vi "GetFirstProcessModule.vi"(7 "originator":string, 8 "error in (no error)":errorcluster, 9 "data":T2, 10 "type":T1, 11 "Qbus in":refnum<class "Qbus.lvclass">) -> (0 "error out":errorcluster, 3 "Qbus out":refnum<class "Qbus.lvclass">)   [LabVIEW 2017, in "DataFlow.lvlib"]
doc: "Sends a data set to the first process in the Dataflow Script via a ProcessDataFlowBlock Qbus message. The first process operates on the data and then transfers it to the next process."
uses:
  <vilib>/addons/InsightCM/Devices/Shared/Common/DataFlow/DataFlow.lvlib
  <vilib>/addons/Qbus/Qbus.lvclass
  <vilib>/addons/InsightCM/Devices/Shared/Common/DataFlow/controls/Data.ctl
  <vilib>/addons/InsightCM/Utilities/DataAccessors/controls/wfmSGL_DVR.ctl
  <vilib>/addons/PointValueMap/controls/PointMap.ctl
  <vilib>/addons/InsightCM/Devices/Shared/Common/DataFlow/controls/Type.ctl
  <vilib>/addons/PointValueMap/subVIs/Point_Write_string.vi
  <vilib>/addons/PointValueMap/PointValueMap.lvlib
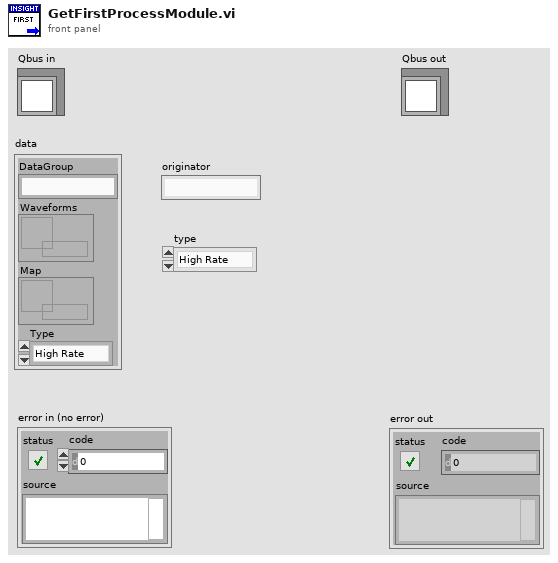
[diagram p1: front panel]
types:
  T1 = typedef "DataFlow.lvlib/Type.ctl" = enum16{"High Rate", "Low Rate", "Burst Mode"}
  T2 = typedef "DataFlow.lvlib/Data.ctl" = cluster{"DataGroup":string, "Waveforms":T3, "Map":T4, "Type":T1}
  T3 = typedef "wfmSGL_DVR.ctl" = refnum<data-value>
  T4 = typedef "PointValueMap.lvlib/PointMap.ctl" = refnum<data-value>
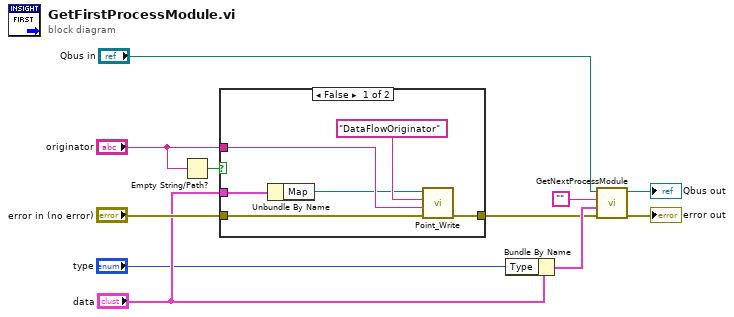
[diagram p0: block diagram]
diagram:
  n1 = Empty String/Path?(string/path="originator") -> (empty?=w2:bool)
  n2 = case shown="False" w2 {
    tunnel: "originator" -> [w17 _]
    tunnel: "error in (no error)" -> [w15 w18]
    tunnel: [w14 w18] -> w5
    tunnel: "data" -> [w13 _]
    frame False {
      n3 = Unbundle By Name(w13) -> ("Map"=w12:T4)
      n4 = call-poly <vilib>:"Point_Write.vi"("Error In"=w15, "Value"=w17, "Tag"="DataFlowOriginator", "Map"=w12) -> ("Error Out"=w14:errorcluster)  [unwired: 6 in, 1 out]
    }
    frame True {
    }
  }
  n5 = Bundle By Name(cluster="data", "Type"="type") -> (w7:T2)
  n6 = call <vilib>:"GetNextProcessModule.vi"("error in (no error)"=w5, "data"=w7, "source"="", "Qbus in"="Qbus in") -> ("error out"=→"error out":errorcluster, "Qbus out"=→"Qbus out":refnum<class "Qbus.lvclass">)  [unwired: 6 in]
